vi "Test Set Symbol.vi"(8 "error in (no error)":errorcluster, 11 "Test Case In":refnum<class "Conditional Disabled Configurator Test.lvclass">) -> (0 "error out":errorcluster, 3 "Test Case Out":refnum<class "Conditional Disabled Configurator Test.lvclass">)   [LabVIEW 2020, in "Conditional Disabled Configurator Test.lvclass"]
uses:
  Conditional Disabled Configurator Test.lvclass
  Conditional Disabled Configurator Test.lvclass/Conditional Disabled Configurator Test.ctl
  01074fa8-ee8a-411d-bc8b-fc92c4f90959.vi
  source/Conditional Disabled Configurator/Conditional Disabled Configurator.lvclass
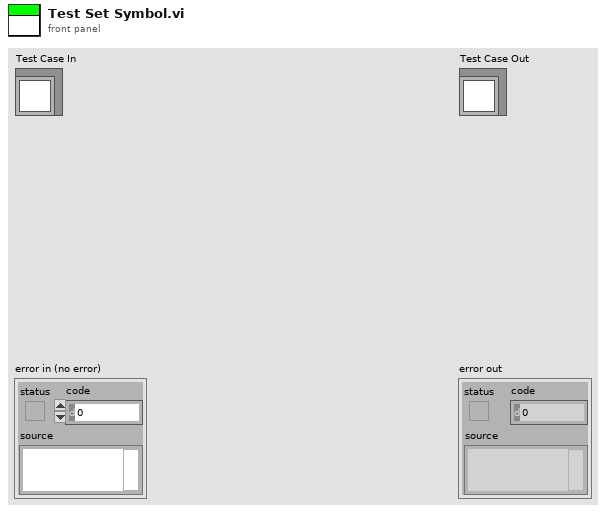
[diagram p1: front panel]
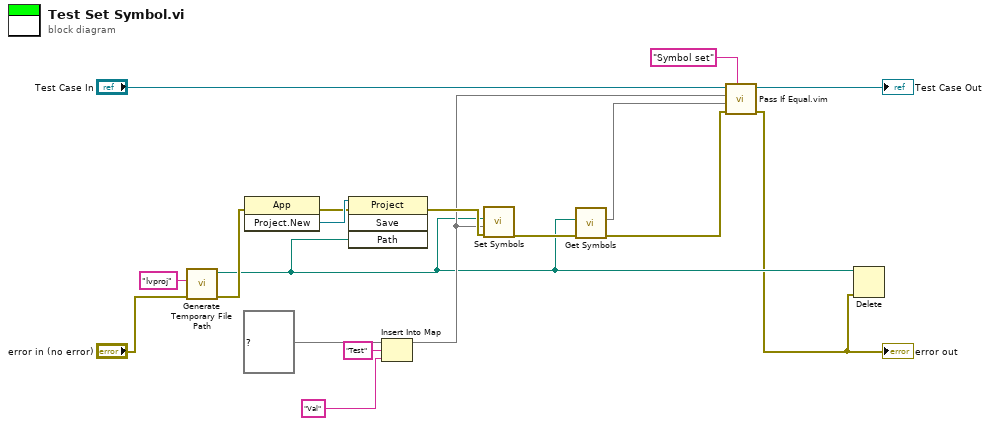
[diagram p0: block diagram]
diagram:
  n1 = call <vilib>:"Generate Temporary File Path.vi"("error in (no error)"="error in (no error)", "Temporary File Extension (tmp)"="lvproj") -> ("error out"=w14:errorcluster, "Unique Temporary File Path"=w2:path)  [unwired: 8 in]
  n2 = invoke class="App" method="Project.New"(error in=w14) -> (error out=w12:errorcluster, "Project:New"=w13:refnum<vi>)  [unwired: 2 in, 1 out]
  n3 = invoke class="Project" method="Save"(reference=w13, error in=w12, "Path"=w2) -> (error out=w11:errorcluster)  [unwired: 1 in, 3 out]
  n4 = Insert Into Map(map in=map{string, string} {} ("Symbols"), key="Test", value="Val") -> (map out=w4:map{string, string})  [unwired: 2 out]
  n5 = call "Set Symbols.vi"("error in (no error)"=w11, "Symbols"=w4, "Project Path"=w2) -> ("error out"=w7:errorcluster)  [unwired: 8 in]
  n6 = call "Get Symbols.vi"("error in (no error)"=w7, "Project Path"=w2) -> ("error out"=w5:errorcluster, "Symbols"=w6:map{string, string})  [unwired: 8 in]
  n7 = call "Pass If Equal.vim"("Description"="Symbol set", "error in (no error)"=w5, "Actual"=w6, "Expected"=w4, "LUnit Test Case In"="Test Case In") -> ("error out"=w1:errorcluster, "LUnit Test Case Out"=→"Test Case Out":refnum<class "Conditional Disabled Configurator Test.lvclass">)  [unwired: 5 in]
  "error out" <- w1
  n8 = Delete(path (use dialog)=w2, error in=w1) -> ()  [unwired: 3 in, 3 out]
